vi "FileIO-File or Folder Exists.vi"(8 "error in (no error)":errorcluster, 9 "extension":string="*", 11 "path":path) -> (0 "error out":errorcluster, 1 "Exists?":bool, 2 "Directory?":bool, 3 "dup path":path)   [LabVIEW 2020]
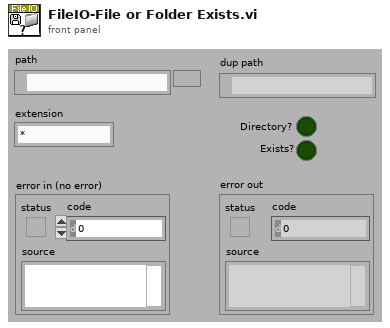
[diagram p1: front panel]
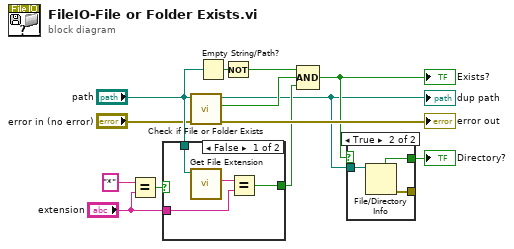
[diagram p0: block diagram]
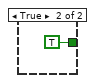
[diagram p3: hidden frame]
diagram:
  n1 = Equal?(x="*", y="extension") -> (x = y?=w6:bool)
  n2 = case shown="False" w6 {
    tunnel: "extension" -> [w16 _]
    tunnel: [w15 TRUE] -> w9
    tunnel: "path" -> [w14 _]
    frame False {
      n3 = call <vilib>:"Get File Extension.vi"("file"=w14) -> ("lowercase file extension"=w17:string)  [unwired: 6 in, 4 out]
      n4 = Equal?(x=w17, y=w16) -> (x = y?=w15:bool)
    }
    frame True {
    }
  }
  n5 = call <vilib>:"Check if File or Folder Exists.vi"("error in (no error)"="error in (no error)", "path"="path") -> ("error out"=→"error out":errorcluster, "file or folder exists?"=w12:bool, "dup path"=w2:path)  [unwired: 7 in]
  "dup path" <- w2
  n6 = Empty String/Path?(string/path="path") -> (empty?=w11:bool)
  n7 = Not(x=w11) -> (.not. x?=w10:bool)
  n8 = Compound Arithmetic op=AND(w10, w12, w9) -> (w3:bool)
  "Exists?" <- w3
  n9 = case shown="True" w3 {
    tunnel: w2 -> [_ w21]
    tunnel: [_ w20] -> _
    tunnel: [_ w19] -> w1
    frame False {
    }
    frame True {
      n10 = File/Directory Info(path=w21) -> (directory=w19:bool, error out=w20:errorcluster)  [unwired: 1 in, 5 out]
    }
  }
  "Directory?" <- w1
